vi "process.vi"(8 "error in (no error)":errorcluster, 10 "Process":string, 11 "Thermocouples in":refnum<class "Thermocouples.lvclass">) -> (0 "error out":errorcluster, 2 "Variant":variant, 3 "Thermocouples out":refnum<class "Thermocouples.lvclass">)   [LabVIEW 2025, in "Thermocouples.lvclass"]
uses:
  Thermocouples.lvclass
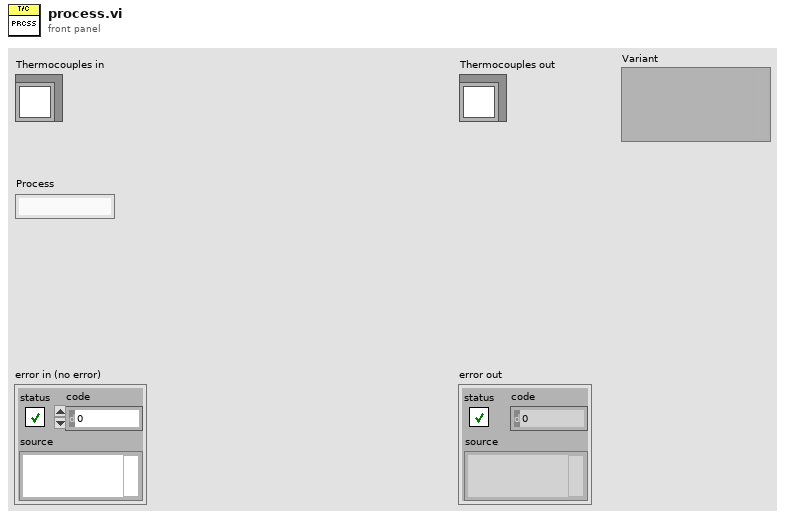
[diagram p1: front panel]
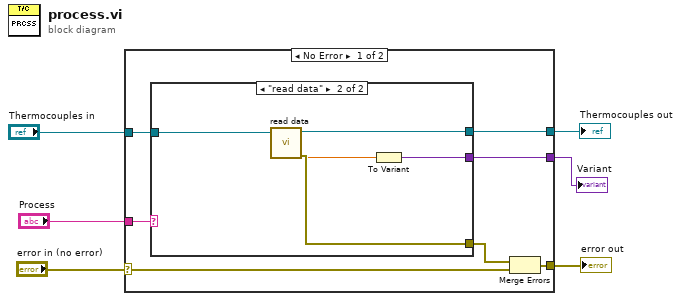
[diagram p0: block diagram]
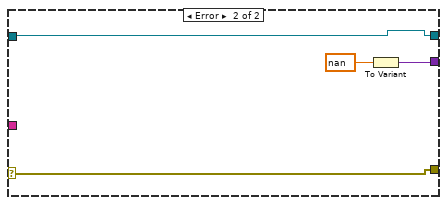
[diagram p3: hidden frame]
diagram:
  n1 = case shown="No Error" "error in (no error)" {
    selector: "error in (no error)" -> [w8 w22]
    tunnel: "Process" -> [w13 _]
    tunnel: "Thermocouples in" -> [w12 w23]
    tunnel: [w11 w23] -> w3
    tunnel: [w10 w22] -> w2
    tunnel: [w7 w20] -> w1
    frame No Error {
      n2 = case shown="\"read data\"" w13 {
        tunnel: w12 -> [w14 w19]
        tunnel: [w14 w18] -> w11
        tunnel: [_ w17] -> w9
        tunnel: [_ w15] -> w7
        frame "False", Default {
        }
        frame "read data" {
          n3 = call-dynamic "read data.vi"("Thermocouples in"=w19) -> ("error out"=w17:errorcluster, "data"=w16:dbl, "Thermocouples out"=w18:refnum<class "Thermocouples.lvclass">)  [unwired: 8 in]
          n4 = To Variant(anything=w16) -> (Variant=w15:variant)
        }
      }
      n5 = Merge Errors(w9, w8) -> (w10:errorcluster)
    }
    frame Error {
      n6 = To Variant(anything=nan ("data")) -> (Variant=w20:variant)
    }
  }
  "error out" <- w2
  "Thermocouples out" <- w3
  "Variant" <- w1
